vi "Get Call Registration.vi"(8 "error in (no error)":errorcluster, 11 "Node in":refnum<class "PyObject.lvclass">) -> (0 "error out":errorcluster, 2 "Call Registration":T1, 3 "Node out":refnum<class "PyObject.lvclass">)   [LabVIEW 2015, in "JKI_Python_Bridge_for_LV.lvlib" / "PyObject.lvclass"]
uses:
  PyObject.lvclass
  Server/Type Definitions/Python Method Call - Event Registration.ctl
  Call/Call.lvclass
  Server/Type Definitions/Public Events - Cluster.ctl
  PyObject.lvclass/PyObject.ctl
  Server/Server.lvclass
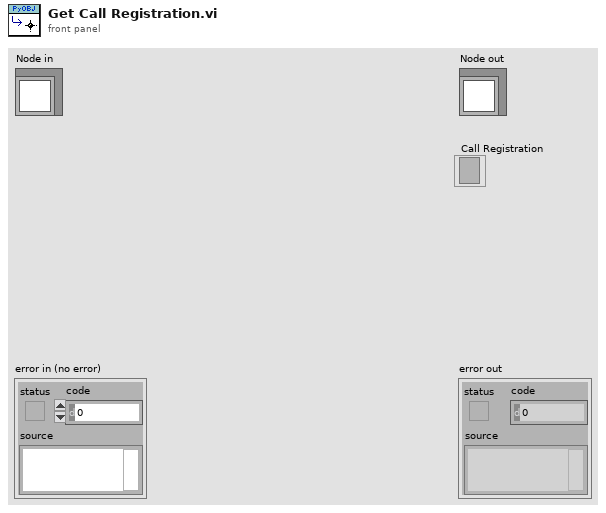
[diagram p1: front panel]
types:
  T1 = typedef "JKI_Python_Bridge_for_LV.lvlib/Server.lvclass/Python Method Call - Event Registration.ctl" = refnum<event-registration>
  T2 = typedef "JKI_Python_Bridge_for_LV.lvlib/PyObject.lvclass/Private Data.ctl" = cluster{"Call Registration":T1, "Functions":T3[], "Object Name":string}
  T3 = typedef "JKI_Python_Bridge_for_LV.lvlib/PyObject.lvclass/PyObject Method.ctl" = cluster{"Name":string, "Arguments":string[], "Documentation":string}
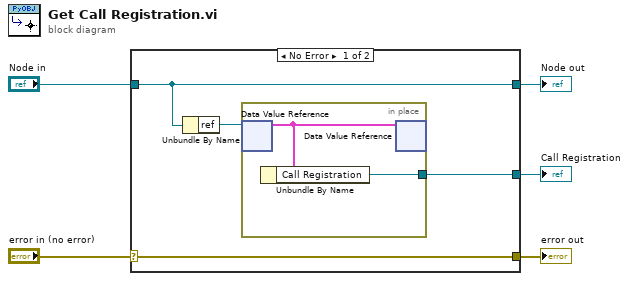
[diagram p0: block diagram]
diagram:
  n1 = case shown="No Error" "error in (no error)" {
    selector: "error in (no error)" -> [w9 w12]
    tunnel: [w9 w12] -> w4
    tunnel: [w8 w13] -> w2
    tunnel: "Node in" -> [w8 w13]
    tunnel: [w6 _] -> w1
    frame No Error {
      n2 = Unbundle By Name(w8) -> ("ref"=w7:refnum<data-value>)
      n3 = in-place {
        in-place-border: [w10] -> w6
        n4 = in-place-dvr #1(w7) -> (w11:T2)  [unwired: 1 out]
        n5 = Unbundle By Name(w11) -> ("Call Registration"=w10:T1)
        n6 = in-place-dvr #1(w11) -> ()  [unwired: 2 out]
      }
    }
    frame Error {
    }
  }
  "error out" <- w4
  "Node out" <- w2
  "Call Registration" <- w1
